vi "Treat variables.vi"(0 "Analog Variable info fixed":T3[](array[typedef]) {"Default Scaling"."Offset" format="%.5f"; "Default Scaling"."Gain" format="%.5f"}, 5 "Common alarm handling(F)":bool, 7 "Analog values":dbl[](array[numeric]), 9 "Variabel start index":i32, 11 "error In":errorcluster, 12 "Analog Variable info Settings":T9[](array[typedef]) {"Scaling"."Offset" format="%.5f"; "Scaling"."Gain" format="%.5f"; "Limits and responces"."Limits"."H" format="%.3f"; "Limits and responces"."Limits"."L" format="%.3f"; "Limits and responces"."Limits"."HH" format="%.3f"; "Limits and responces"."Limits"."LL" format="%.3f"}) -> (3 "Catagorised  Stsaus":T1[](array[typedef]), 4 "Analog Variable Display":T14[](array[typedef]) {"Value" format="%#.1f"}, 6 "Action":T12, 8 "Analog Values":dbl[](array[numeric]), 10 "Alarms":bool[](array[boolean]), 15 "error out":errorcluster)   [LabVIEW 2011]
uses:
  Action List.ctl
  GUI/Analog Var Disp 0 sif.ctl
  GUI/Status indicator Black Small.ctl
  User Setting Analog Channel Bg.ctl
  Scaling.ctl
  Alarm Setup Analog.ctl
  Alarm Responce.ctl
  Limits.ctl
  Fixed Analog Channel Definition.ctl
  Units/Quantity enum.ctl
  Update frequensies.ctl
  Channel catagory Enum.ctl
  Channel Classification Enum.ctl
  Catagorised alarm state.ctl
  GUI/Status Indikator Helper.ctl
  Application Structure/Options/Action GFV Settings.ctl
  emi cndiates/E&S/reate/S&E Analog Alarm type.ctl
  emi Lib/System 01/0 - General/emi_Read System ID.vi
  <vilib>/Utility/VariantDataType/GetNumericInfo.vi
  emi Lib/System 01/0 - General/Private/_emi_GFV System ID.vi
  emi Lib/System 01/0 - General/S&E reporting/Private/_emi_S&E Q Generator.vi
  <vilib>/Utility/error.llb/Clear Errors.vi
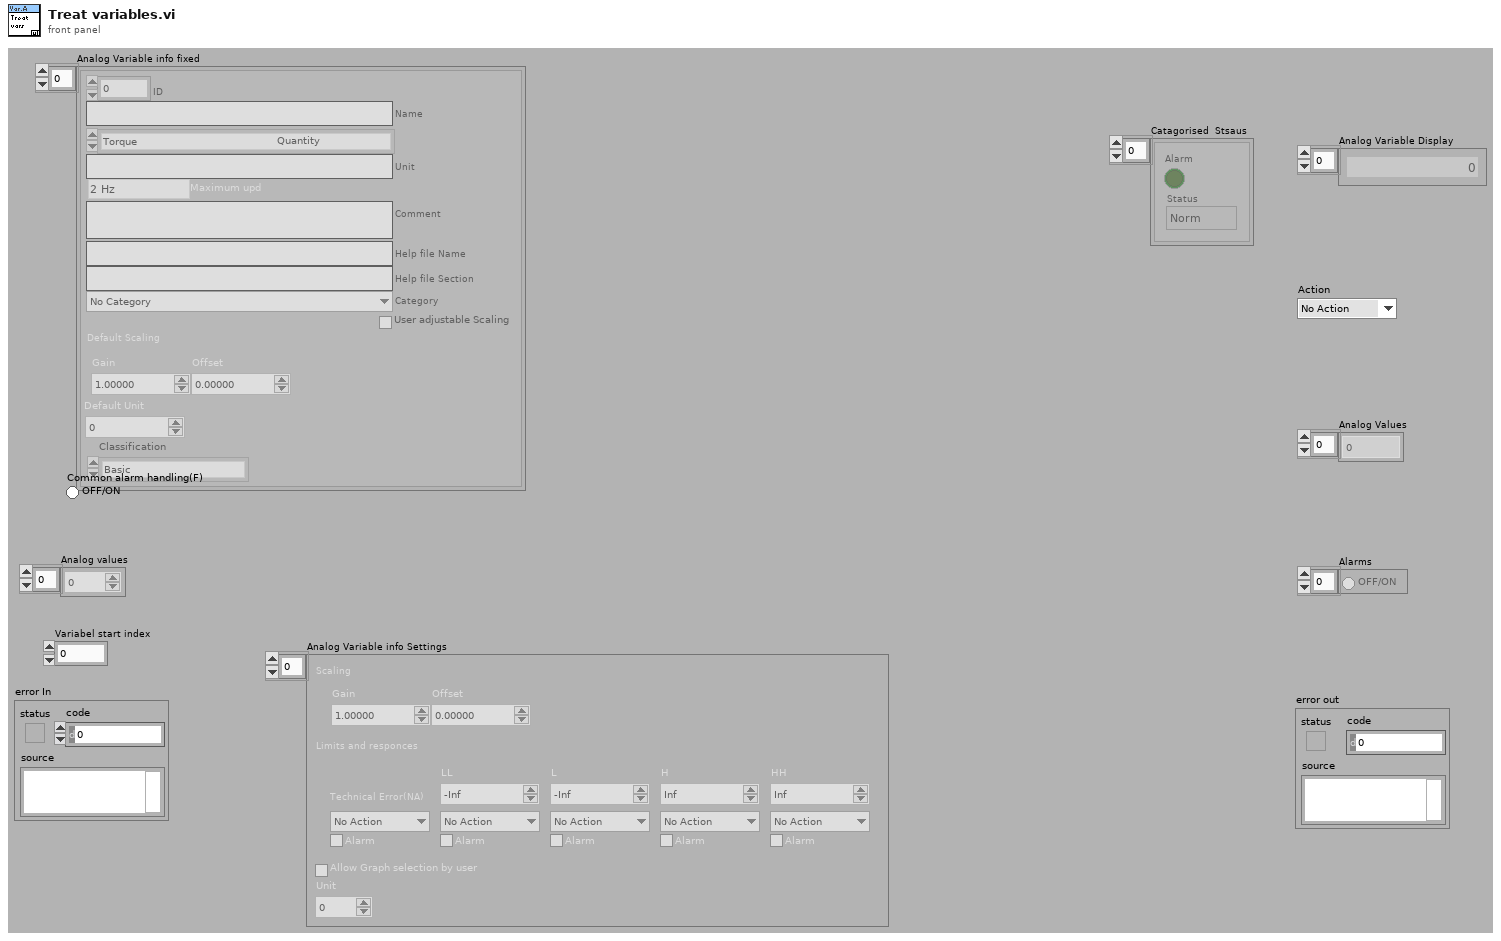
[diagram p1: front panel]
types:
  T1 = typedef "Catagorised alarm state.ctl" = cluster{"Alarm":bool, "Status":T2}
  T2 = typedef "Status Indikator Helper.ctl" = enum16{"Norm", "L", "H", "LL", "HH", "Value", "Technical"}
  T3 = typedef "Fixed Analog Channel Definition.ctl" = cluster{"ID":u16, "Name":string, "Quantity":T4, "Unit":string, "Maximum upd":T5, "Comment":string, "Help file Name":string, "Help file Section ":string, "Category":T6, "User adjustable Scaling":bool, "Default Scaling":T7, "Default Unit":i32, "Classification":T8}
  T4 = typedef "Quantity enum.ctl" = enum16{"NA", "Acceleration", "Angle", "Current", "Force", "Distance", "Pressure", "Resistance", "Rotational Speed", "Speed", "Temperature", "Tension", "Torque", "Voltage", "Weight"}
  T5 = typedef "Update frequensies.ctl" = enum16{"2 Hz", "1 Hz", "0.1 Hz"}
  T6 = typedef "Channel catagory Enum.ctl" = enum16{"No Category", "Power", "Temperature", "Pressure"}
  T7 = typedef "Scaling.ctl" = cluster{"Gain":dbl, "Offset":dbl}
  T8 = typedef "Channel Classification Enum.ctl" = enum16{"Basic", "Advanced", "Expert", "Unused"}
  T9 = typedef "User Setting Analog Channel Bg.ctl" = cluster{"Scaling":T7, "Limits and responces":T10, "Allow Graph selection by user":bool, "Unit":u16}
  T10 = typedef "Alarm Setup Analog.ctl" = cluster{"Technical Error(NA)":T11, "LL":T11, "L":T11, "H":T11, "HH":T11, "Limits":T13}
  T11 = typedef "Alarm Responce.ctl" = cluster{"Action":T12, "Alarm":bool}
  T12 = typedef "Action List.ctl" = enum16{"No Action", "Stop Motor", "Turn Off HV"}
  T13 = typedef "Limits.ctl" = cluster{"LL":dbl, "L":dbl, "H":dbl, "HH":dbl}
  T14 = typedef "Analog Var Disp 0 sif.ctl" = cluster{"Value":dbl, "Unit":string, "Status":T15}
  T15 = typedef "Status indicator Black Small.ctl" = u16
  T16 = typedef "Action GFV Settings.ctl" = enum16{"Init", "Get From INI", "Put In INI", "Get Settings", "Get Update Index", "Set Setting"}
  T17 = typedef "Options  All pages and custom.ctl" = cluster{"P 1 (App)":T18, "P 2":T19, "P 3":T20, "P 4":T23, "P 5":T28, "P 6 (Err)":T29, "P 7 (Expert)":T30, "P 8 (Depth)":T32, "C 1":T33, "C 2":T34}
  T18 = typedef "Options Page 1 (App).ctl" = cluster{"Result files":path, "PCP Interface":string, "Tractor/Stroker Interface":string, "Tractor Interface":string, "Modem Status Interface":string, "Audible Alarm":bool, "Force alarm on Technical":bool, "Force alarm on HH":bool, "Force alarm on LL":bool, "Force alarm on H":bool, "Force alarm on L":bool}
  T19 = typedef "Options Page 2.ctl" = cluster{"Solenoid & Relay latching time":u16, "Tractor relay 1":dbl, "Tractor relay 2":dbl, "Tractor Solenoid limit":dbl}
  T20 = typedef "Options Page 3.ctl" = cluster{"Min resistance":dbl, "Max resistance":dbl, "Head voltage range":T21, "Max voltage jump":dbl, "Maximum resistance change":dbl, "Start Telemetry Voltage":dbl, "Start Telemetry Timeout":dbl, "Start Motor Voltage":dbl, "Stop Motor Voltage":dbl, "Pass Mode Warning Voltage":dbl, "Relay Switch Voltage":dbl, "Relay Status Loss Voltage":dbl, "Samples to average":i32, "PSU type DO NOT USE":T22, "Magna OVP":dbl, "Magna Current Limit":dbl}
  T21 = typedef "PCP type List.ctl" = enum16{"0 - 350V", "0 - 450V", "0 - 600V"}
  T22 = typedef "PSU Type.ctl" = enum16{"Unipower", "Magna 8.3A", "Magna 12A", "None"}
  T23 = typedef "Options Page 4.ctl" = cluster{"Solenoid & Relay latching time":u16, "Stroker relay 1":dbl, "Stroker Relay 2":dbl, "Stroker Solenoid limit":dbl, "Force det.":T24, "Stroke force lim.":dbl, "Anchor Enabled Pressure":dbl, "Tacometer puls":dbl, "Default anchor behavior":T25, "Default stroker behavior":T26, "Default stroker force limit (tonne)":dbl, "Slips Size":T27}
  T24 = typedef "Stroke force selector.ctl" = enum16{"Stroke in = node 1", "Strok out = node 1"}
  T25 = typedef "Default anchor behavior.ctl" = enum16{"Do nothing", "Set Anchor", "Release Anchor"}
  T26 = typedef "Default stroker behavior.ctl" = enum16{"Do nothing", "Stop", "Go Out", "Go In"}
  T27 = typedef "Slips Type Radio.ctl" = enum32{"No Selection", "338 MRS", "3,9 MRS"}
  T28 = typedef "Options Page 5.ctl" = cluster{"Solenoid & Relay latching time":u16, "Driller relay 1":dbl, "Driller Relay 2":dbl, "Driller  Solenoid limit":dbl}
  T29 = typedef "Options Page 6 (Err).ctl" = cluster{"Error and event files":path}
  T30 = typedef "Options Page 7 (Expert).ctl" = cluster{"Show Debug":bool, "Log debug messages":bool, "Additional debug messages":bool, "Start Beagle with Simulator data":bool, "Workshop mode":bool, "Modem baud":u16, "enumCANCOM":bool, "Modem sim":T31, "Telemetry Timeout Disable":i32, "Buffer size":i32, "Upd regular data":bool, "Cable comp":cluster{"VMOD1 Voltage(V)":dbl, "VMOD2 Voltage(V)":dbl}}
  T31 = typedef "Modem simulation setup.ctl" = cluster{"Modem dealay sim":bool, "Sim baud Tx":u16, "Bit Error fraction Tx":dbl, "Sim baud Rx":u16, "Bit Error fraction Rx":dbl}
  T32 = typedef "Options Page 8 (Depth).ctl" = cluster{"Winch Spool Circumference":dbl, "Winch Pulses per Revolution":dbl, "Current Depth":dbl}
  T33 = typedef "Options Custom 1.ctl" = cluster{"Depth Updated":bool, "Depth Offset":dbl}
  T34 = typedef "Options Custom 2.ctl" = cluster{"Placeholder":bool}
  T35 = typedef "S&E Analog Alarm type.ctl" = cluster{"Alarm":bool, "State":T2, "Value":dbl, "Source name":string}
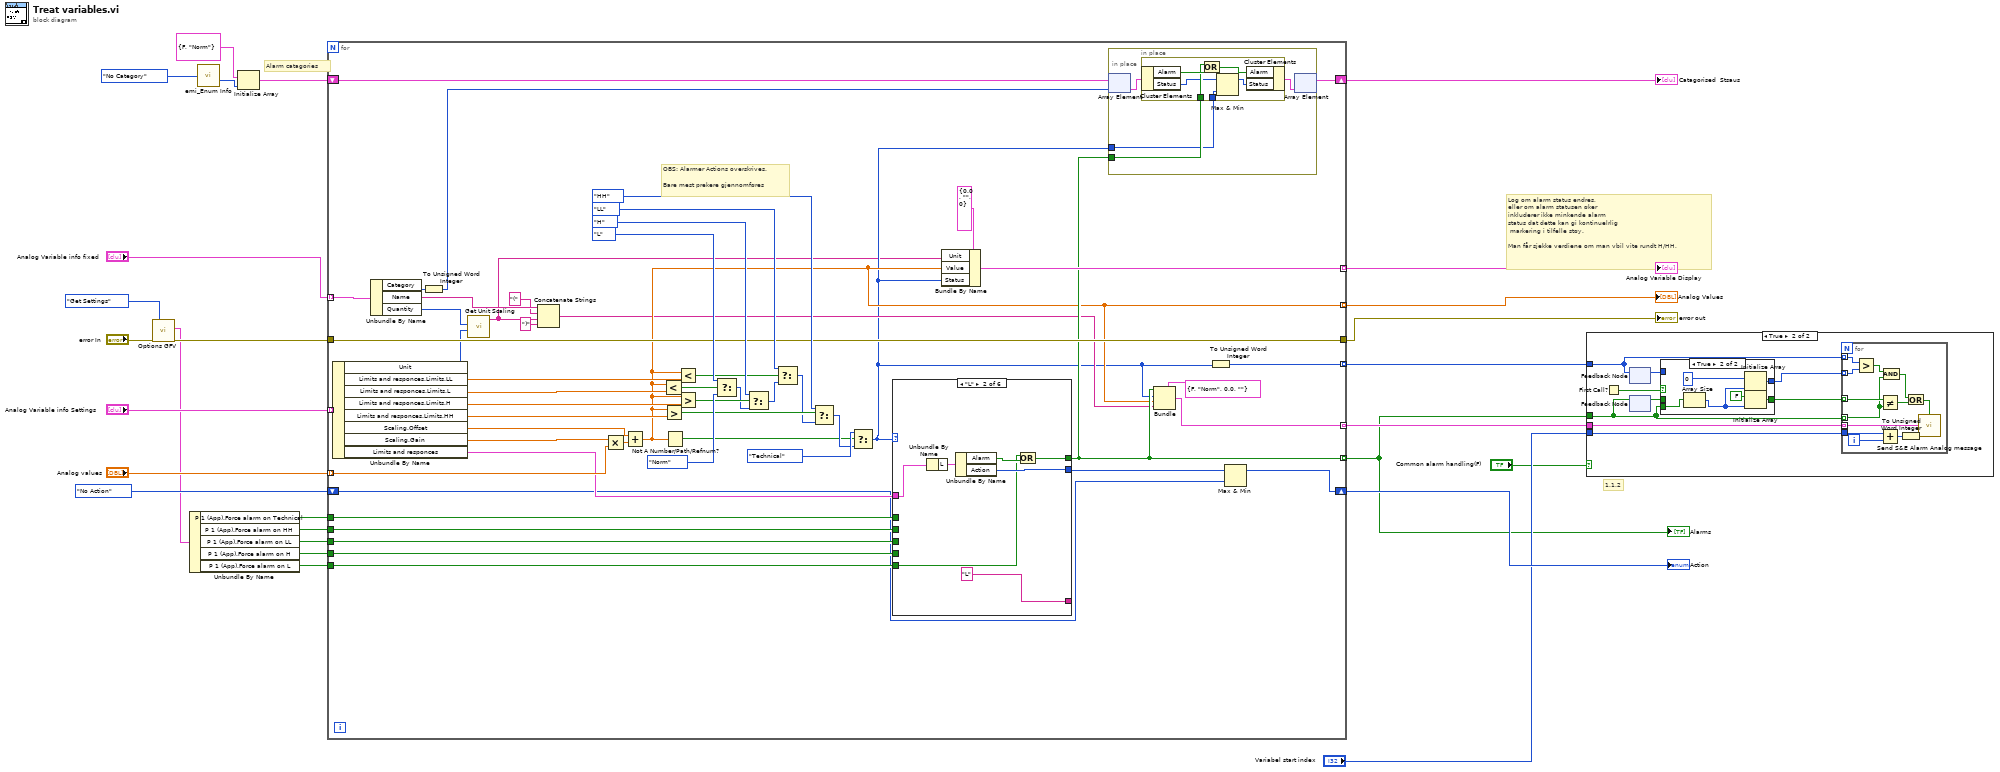
[diagram p0: block diagram]
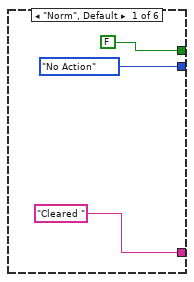
[diagram p4: hidden frame]
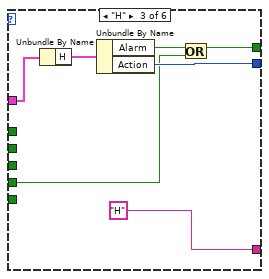
[diagram p5: hidden frame]
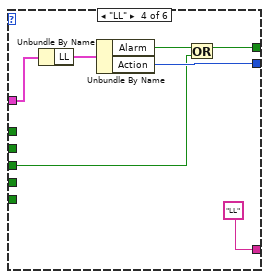
[diagram p6: hidden frame]
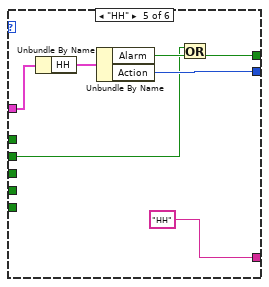
[diagram p7: hidden frame]
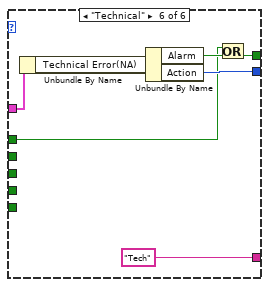
[diagram p8: hidden frame]
diagram:
  # "1.1.2"
  # "Log om alarm status endres, \neller om alarm statusen øker\ninkluderer ikke minkende alarm \nstatus dat dette kan gi kontinuelrlig\n markering i tilfelle støy.\n\nMan får sjekke verdiene om man vbil vite rundt H/HH,"
  # "Alarm catagories"
  n1 = call "Options GFV.vi"("error in (no error)"="error In", "Action(Get Settings)"=Action_GFV_Settings."Get Settings") -> ("Options"=w16:T17, "error out"=w18:errorcluster)  [unwired: 15 in, 1 out]
  n2 = Unbundle By Name(w16) -> ("P 1 (App).Force alarm on Technical"=w15:bool, "P 1 (App).Force alarm on HH"=w14:bool, "P 1 (App).Force alarm on LL"=w13:bool, "P 1 (App).Force alarm on H"=w12:bool, "P 1 (App).Force alarm on L"=w11:bool)
  n3 = call "emi_Enum Info.vi"("Enum"=Channel_catagory_Enum."No Category" ("Catagory")) -> ("Numb Elements"=w6:i32)  [unwired: 11 in, 3 out]
  n4 = Initialize Array(T1 {"Alarm"=FALSE, "Status"=enum."Norm"} ("catagori"), w6) -> (w4:T1[])
  n5 = for {
    tunnel: "Analog values" -> [w77] mode=indexing
    tunnel: "Analog Variable info Settings" -> [w56] mode=indexing
    tunnel: "Analog Variable info fixed" -> [w81] mode=indexing
    tunnel: w18 -> [w53]
    tunnel: [w40] -> w2 mode=indexing
    tunnel: [w54] -> w23 mode=indexing
    tunnel: [w53] -> w24
    tunnel: [w39] -> w10 mode=indexing
    shift-right: [w51] -> w27
    shift-left: Action_List."No Action" ("Action") -> [w28]
    tunnel: w15 -> [w45]
    tunnel: w14 -> [w46]
    tunnel: w13 -> [w47]
    tunnel: w12 -> [w48]
    tunnel: w11 -> [w49]
    tunnel: [w37] -> w9 mode=indexing
    tunnel: [w35] -> w7 mode=indexing
    shift-right: [w33] -> w3
    shift-left: w4 -> [w34]
    # "OBS: Alarmer Actions overskrives.\n\nBare mest prekere gjennomføres"
    n6 = Unbundle By Name(w56) -> ("Unit"=w31:u16, "Limits and responces.Limits.LL"=w73:dbl, "Limits and responces.Limits.L"=w74:dbl, "Limits and responces.Limits.H"=w72:dbl, "Limits and responces.Limits.HH"=w71:dbl, "Scaling.Offset"=w75:dbl, "Scaling.Gain"=w78:dbl, "Limits and responces"=w55:T10)
    n7 = Unbundle By Name(w81) -> ("Category"=w50:T6, "Name"=w44:string, "Quantity"=w29:T4)
    n8 = To Unsigned Word Integer(number=w50) -> (unsigned 16bit integer=w32:u16)
    n9 = call "Get Unit Scaling.vi"("Unit Index"=w31, "Quantity"=w29) -> ("Unit"=w30:string)  [unwired: 7 in, 2 out]
    n10 = Concatenate Strings(w44, "(" ("string"), w30, ")" ("string")) -> (w38:string)
    n11 = Multiply(x=w78, y=w77) -> (x*y=w76:dbl)
    n12 = Add(x=w75, y=w76) -> (x+y=w39:dbl)
    n13 = Less?(x=w39, y=w74) -> (x < y?=w69:bool)
    n14 = Greater?(x=w39, y=w71) -> (0:w61:bool)
    n15 = Not A Number/Path/Refnum?(number/path/refnum=w39) -> (NaN/Path/Refnum?=w57:bool)
    n16 = Less?(x=w39, y=w73) -> (x < y?=w63:bool)
    n17 = Greater?(x=w39, y=w72) -> (0:w67:bool)
    n18 = Select(t=Status_Indikator_Helper."L" ("Enum"), s=w69, f=Status_Indikator_Helper."Norm" ("Enum")) -> (s? t:f=w66:T2)
    n19 = Select(t=Status_Indikator_Helper."H" ("Enum"), s=w67, f=w66) -> (s? t:f=w64:T2)
    n20 = Select(t=Status_Indikator_Helper."LL" ("Enum"), s=w63, f=w64) -> (s? t:f=w59:T2)
    n21 = Select(t=Status_Indikator_Helper."HH" ("Enum"), s=w61, f=w59) -> (s? t:f=w58:T2)
    n22 = Select(t=Status_Indikator_Helper."Technical" ("Enum"), s=w57, f=w58) -> (s? t:f=w36:T2)
    n23 = case shown="\"L\"" w36 {
      tunnel: w55 -> [_ w101 w108 w115 w122 w129]
      tunnel: [Action_List."No Action" ("LL.Action") w98 w105 w112 w119 w126] -> w52
      tunnel: [FALSE w97 w104 w111 w118 w125] -> w40
      tunnel: w49 -> [_ w96 _ _ _ _]
      tunnel: w48 -> [_ _ w103 _ _ _]
      tunnel: w47 -> [_ _ _ w110 _ _]
      tunnel: w46 -> [_ _ _ _ w117 _]
      tunnel: w45 -> [_ _ _ _ _ w124]
      tunnel: ["Cleared " "L" "H" "LL" "HH" "Tech"] -> _
      frame "Norm", Default {
      }
      frame "L" {
        n24 = Unbundle By Name(w101) -> ("L"=w100:T11)
        n25 = Unbundle By Name(w100) -> ("Alarm"=w99:bool, "Action"=w98:T12)
        n26 = Or(x=w96, y=w99) -> (x .or. y?=w97:bool)
      }
      frame "H" {
        n27 = Unbundle By Name(w108) -> ("H"=w107:T11)
        n28 = Unbundle By Name(w107) -> ("Alarm"=w106:bool, "Action"=w105:T12)
        n29 = Or(x=w106, y=w103) -> (x .or. y?=w104:bool)
      }
      frame "LL" {
        n30 = Unbundle By Name(w115) -> ("LL"=w114:T11)
        n31 = Unbundle By Name(w114) -> ("Alarm"=w113:bool, "Action"=w112:T12)
        n32 = Or(x=w113, y=w110) -> (x .or. y?=w111:bool)
      }
      frame "HH" {
        n33 = Unbundle By Name(w122) -> ("HH"=w121:T11)
        n34 = Unbundle By Name(w121) -> ("Alarm"=w120:bool, "Action"=w119:T12)
        n35 = Or(x=w117, y=w120) -> (x .or. y?=w118:bool)
      }
      frame "Technical" {
        n36 = Unbundle By Name(w129) -> ("Technical Error(NA)"=w128:T11)
        n37 = Unbundle By Name(w128) -> ("Alarm"=w127:bool, "Action"=w126:T12)
        n38 = Or(x=w124, y=w127) -> (x .or. y?=w125:bool)
      }
    }
    n39 = Bundle By Name(cluster=T14 {"Value"=0.0, "Unit"="", "Status"=0} ("Cluster 4"), "Unit"=w30, "Value"=w39, "Status"=w36) -> (w54:T14)
    n40 = in-place {
      in-place-border: w36 -> [w82]
      in-place-border: w40 -> [w83]
      n41 = in-place-array #1(w34, w32) -> (w85:T1)
      n42 = in-place {
        in-place-border: w83 -> [w89]
        in-place-border: w82 -> [w87]
        n43 = in-place-cluster #2(w85) -> ("Alarm"=w91:bool, "Status"=w88:T2)
        n44 = Or(x=w89, y=w91) -> (x .or. y?=w90:bool)
        n45 = Max & Min(x=w88, y=w87) -> (max(x,y)=w86:u16)  [unwired: 1 out]
        n46 = in-place-cluster #2("Alarm"=w90, "Status"=w86) -> (w84:T1)
      }
      n47 = in-place-array #1(w84) -> (w33:T1[])  [unwired: 1 out]
    }
    n48 = Bundle(cluster=T35 {"Alarm"=FALSE, "State"=enum."Norm", "Value"=0.0, "Source name"=""} ("S&E Alarm"), "Alarm"=w40, "State"=w36, "Value"=w39, "Source name"=w38) -> (w37:T35)
    n49 = To Unsigned Word Integer(number=w36) -> (unsigned 16bit integer=w35:u16)
    n50 = Max & Min(x=w52, y=w28) -> (max(x,y)=w51:u16)  [unwired: 1 out]
  }
  "Action" <- w27
  "Analog Values" <- w10
  "error out" <- w24
  "Alarms" <- w2
  "Analog Variable Display" <- w23
  "Catagorised  Stsaus" <- w3
  n51 = case shown="True" "Common alarm handling(F)" {
    tunnel: w9 -> [_ w138]
    tunnel: "Variabel start index" -> [_ w137]
    tunnel: w7 -> [_ w136]
    tunnel: w2 -> [_ w130]
    frame False {
    }
    frame True {
      n52 = First Call?() -> (First Call?: T/F=w135:bool)
      n53 = feedback #3() -> (w134:u16[])  [unwired: 1 in]
      n54 = feedback-in #3(w136) -> ()
      n55 = feedback #4() -> (w133:bool[])  [unwired: 1 in]
      n56 = feedback-in #4(w130) -> ()
      n57 = case shown="True" w135 {
        tunnel: w134 -> [w153 _]
        tunnel: w133 -> [w152 _]
        tunnel: [w152 w157] -> w132
        tunnel: [w153 w156] -> w131
        tunnel: w130 -> [_ w154]
        frame False {
        }
        frame True {
          n58 = Array Size(array=w154) -> (size(s)=w159:i32)
          n59 = Initialize Array(u16 0 ("unsigned 16bit integer"), w159) -> (w156:u16[])
          n60 = Initialize Array(FALSE, w159) -> (w157:bool[])
        }
      }
      n61 = for {
        tunnel: w132 -> [w151] mode=indexing
        tunnel: w130 -> [w141] mode=indexing
        tunnel: w138 -> [w145] mode=indexing
        tunnel: w137 -> [w148]
        tunnel: w136 -> [w144] mode=indexing
        tunnel: w131 -> [w143] mode=indexing
        i -> [w149]
        n62 = Greater?(x=w144, y=w143) -> (0:w142:bool)
        n63 = Not Equal?(x=w151, y=w141) -> (x != y?=w150:bool)
        n64 = Add(x=w148, y=w149) -> (x+y=w147:i32)
        n65 = And(x=w142, y=w141) -> (x .and. y?=w140:bool)
        n66 = To Unsigned Word Integer(number=w147) -> (unsigned 16bit integer=w146:u16)
        n67 = Or(x=w140, y=w150) -> (x .or. y?=w139:bool)
        n68 = call "Send S&E Alarm Analog message.vi"("Send(T)"=w139, "S&E Alarm"=w145, "Loc Sub ID/Alarm ID"=w146) -> ()  [unwired: 11 in, 2 out]
      }
    }
  }
